vi "Cowl_Execute.vi"() -> ()   [LabVIEW 2020]
uses:
  Cowl_Cluster.ctl
  Cowl_States.ctl
  Utility VIs/Basic_Motor_Modes.ctl
  Globals/Cowl_Globals.vi
  Globals/Sensor_Values.vi
panel:
  in  "Cowl_Lower_Limit":dbl
  in  "Cowl_Upper_Limit":dbl
  out "Cowl_Output":dbl
  in  "Kp":dbl
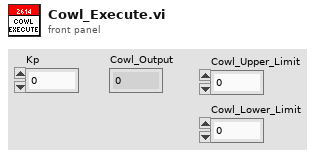
[diagram p1: front panel]
types:
  T1 = typedef "Cowl_Cluster.ctl" = cluster{"Cowl_Control_State":T2, "Manual_Cowl_Throttle":dbl, "Cowl_Goal_Angle":dbl}
  T2 = typedef "Cowl_States.ctl" = enum16{"Manual_%VBus", "GoToAngle", "No-Op"}
  T3 = typedef "Basic_Motor_Modes.ctl" = enum16{"Percent_Voltage", "Speed_Control", "Position_Control", "Current"}
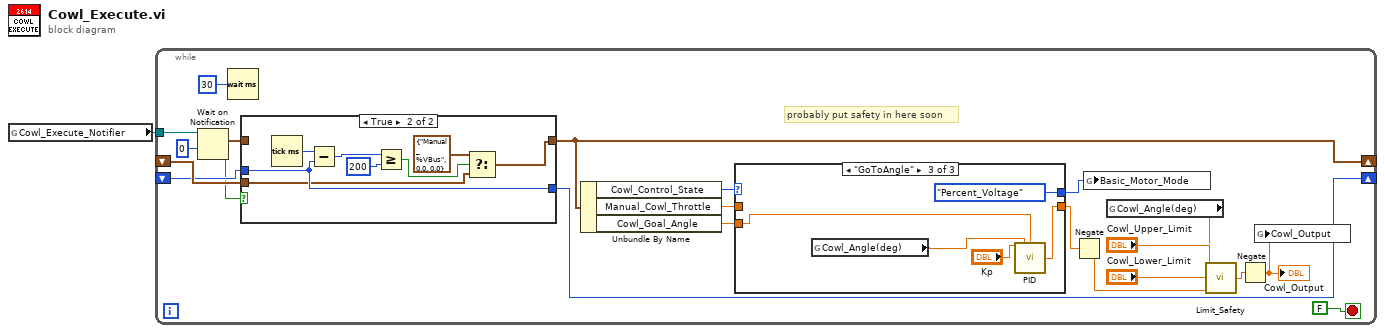
[diagram p0: block diagram]
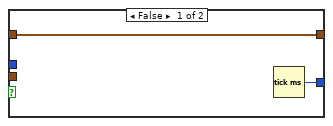
[diagram p2: hidden frame]
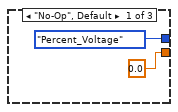
[diagram p3: hidden frame]
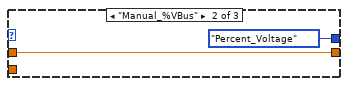
[diagram p4: hidden frame]
diagram:
  n1 = global read "Cowl_Globals.vi" "Cowl_Execute_Notifier"() -> (w1:refnum<notifier>)
  n2 = while {
    tunnel: w1 -> [w20]
    shift-right: [w13] -> _
    shift-left: _ -> [w14]
    shift-right: [w16] -> _
    shift-left: _ -> [w12]
    stop <- FALSE stop-if-true
    # "probably put safety in here soon"
    n3 = Wait on Notification(notifier=w20, timeout in ms (-1)=0) -> (notification=w15:T1, timed out?=w11:bool)  [unwired: 2 in, 2 out]
    n4 = Wait (ms)(milliseconds to wait=u32 30) -> ()  [unwired: 1 out]
    n5 = case shown="True" w11 {
      tunnel: w15 -> [w24 _]
      tunnel: [w24 w27] -> w13
      tunnel: [w23 w31] -> w16
      tunnel: w12 -> [_ w31]
      tunnel: w14 -> [_ w26]
      frame False {
        n6 = Tick Count (ms)() -> (millisecond timer value=w23:u32)
      }
      frame True {
        n7 = Tick Count (ms)() -> (millisecond timer value=w32:u32)
        n8 = Subtract(x=w32, y=w31) -> (x-y=w30:u32)
        n9 = Greater Or Equal?(x=w30, y=u32 200) -> (x >= y?=w28:bool)
        n10 = Select(t=T1 {"Cowl_Control_State"=enum."Manual_%VBus", "Manual_Cowl_Throttle"=0.0, "Cowl_Goal_Angle"=0.0} ("notification"), s=w28, f=w26) -> (s? t:f=w27:T1)
      }
    }
    n11 = Unbundle By Name(w13) -> ("Cowl_Control_State"=w19:T2, "Manual_Cowl_Throttle"=w18:dbl, "Cowl_Goal_Angle"=w6:dbl)
    n12 = case shown="\"GoToAngle\"" w19 {
      tunnel: w18 -> [_ w36 _]
      tunnel: [0.0 ("Command") w36 w41] -> w5
      tunnel: [Basic_Motor_Modes."Percent_Voltage" ("Basic_Motor_Mode") Basic_Motor_Modes."Percent_Voltage" ("Basic_Motor_Mode") Basic_Motor_Modes."Percent_Voltage" ("Basic_Motor_Mode")] -> w17
      tunnel: w6 -> [_ _ w38]
      frame "No-Op", Default {
      }
      frame "Manual_%VBus" {
      }
      frame "GoToAngle" {
        n13 = global read "Sensor_Values.vi" "Cowl_Angle(deg)"() -> (w37:dbl)
        n14 = call "PID.vi"("Kp"="Kp", "Process Variable"=w37, "Goal"=w38) -> ("Command"=w41:dbl)  [unwired: 10 in, 2 out]
      }
    }
    n15 = Negate(x=w5) -> (-x=w4:dbl)
    n16 = global write "Cowl_Globals.vi" "Basic_Motor_Mode"(w17) -> ()
    n17 = global read "Sensor_Values.vi" "Cowl_Angle(deg)"() -> (w7:dbl)
    n18 = call "Limit_Safety.vi"("Outer_Arm_Pivot_Throttle"=w4, "Lower_Limit"="Cowl_Lower_Limit", "Upper_Limit"="Cowl_Upper_Limit", "Sensor_Value"=w7) -> ("Corrected Output"=w3:dbl)  [unwired: 2 in]
    n19 = Negate(x=w3) -> (-x=w2:dbl)
    "Cowl_Output" <- w2
    n20 = global write "Cowl_Globals.vi" "Cowl_Output"(w2) -> ()
  }
